vi "Start.vi"(0 "eye scan in":refnum<class "niHighSpeedSerial Eye Scan v1 Host.lvclass">, 11 "error in":errorcluster) -> (4 "eye scan out":refnum<class "niHighSpeedSerial Eye Scan v1 Host.lvclass">, 15 "error out":errorcluster)   [LabVIEW 2014, in "niHighSpeedSerial Eye Scan v1 Host.lvclass"]
doc: "Moves the session into the Running state and begins measuring the first point.\n\n<B>Input Parameters</B>\n\n<B>eye scan in</B> Takes in a reference to your session from the previous VI.\n\n<B>error in</B> describes error conditions that occur before this node runs. This input provides standard 'error in' functionality.\n\n<B>Output Parameters</B>\n\n<B>eye scan out</B> passes a reference to your session to the next VI.\n\n<B>error out</B> contains error information. This output provides standard 'error out' functionality."
uses:
  <instrlib>/niHighSpeedSerial/Eye Scan/v1/Host/Eye Scan/niHighSpeedSerial Eye Scan v1 Host.lvclass
  <instrlib>/niHighSpeedSerial/Eye Scan/v1/Host/Eye Scan/niHighSpeedSerial Eye Scan v1 Host.lvclass/niHighSpeedSerial Eye Scan v1 Host.ctl
  <instrlib>/niHighSpeedSerial/Eye Scan/v1/Host/Eye Scan/Private/Measure State.ctl
  <vilib>/Utility/error.llb/Error Cluster From Error Code.vi
  <vilib>/ErrorRing/Error Ring.xnode
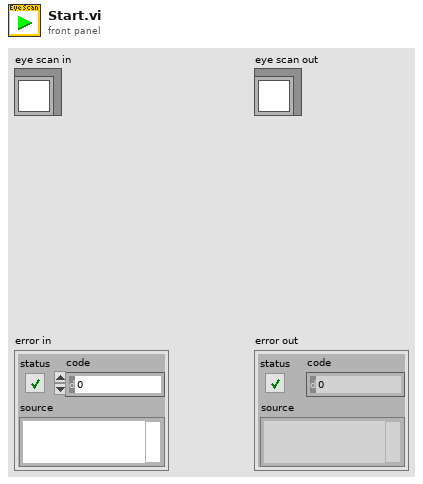
[diagram p1: front panel]
types:
  T1 = typedef "niHighSpeedSerial Eye Scan v1 Host.lvclass/Measure State.ctl" = enum16{"Uninitialized", "Initialized", "Ready", "Measuring", "Finished", "Aborted"}
  T2 = typedef "niHighSpeedSerial Eye Scan v1 Host.lvclass/Private Data.ctl" = cluster{"instruction target":refnum<class "niInstr Instruction Target v1 Host.lvclass">, "channels":T3[], "measure state":T1, "rx output divider":T4, "equalization mode":T5, "rx data width":T6, "BER floor":dbl, "number of points completed":i32, "rx output divider configured?":bool, "equalization mode configured?":bool, "rx data width configured?":bool}
  T3 = typedef "niHighSpeedSerial Eye Scan v1 Host.lvclass/Channel Data.ctl" = cluster{"instance":u8, "channel":refnum<class "niHighSpeedSerial Eye Scan Single Point v1 Host.lvclass">, "point iterator":refnum<class "niHighSpeedSerial Eye Scan Point Iterator v1 Host.lvclass">}
  T4 = typedef "niHighSpeedSerial Eye Scan Common v1 Host.lvlib/RX Output Divider.ctl" = enum16{"1", "2", "4", "8", "16"}
  T5 = typedef "niHighSpeedSerial Eye Scan Common v1 Host.lvlib/Equalization Mode.ctl" = enum16{"DFE", "LPM"}
  T6 = typedef "niHighSpeedSerial Eye Scan Common v1 Host.lvlib/Data Width.ctl" = enum16{"16 Bit", "20 Bit", "32 Bit", "40 Bit"}
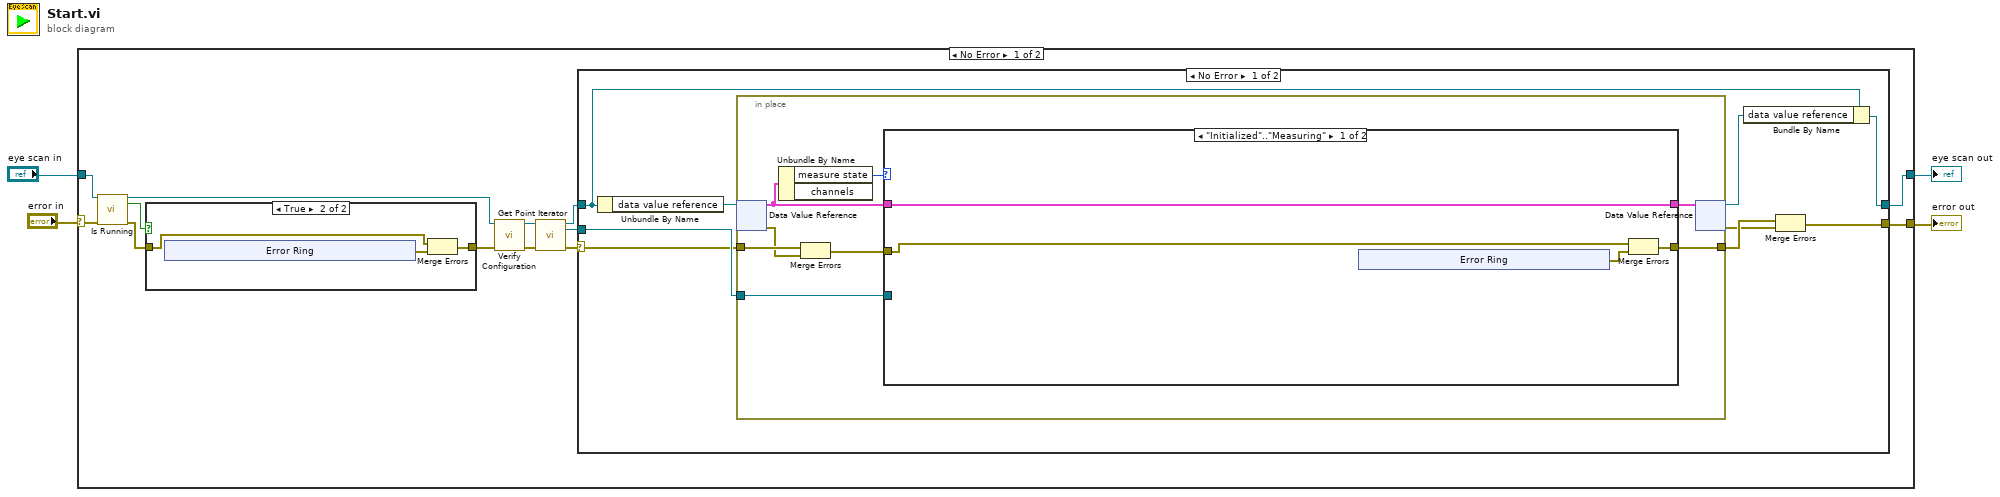
[diagram p0: block diagram]
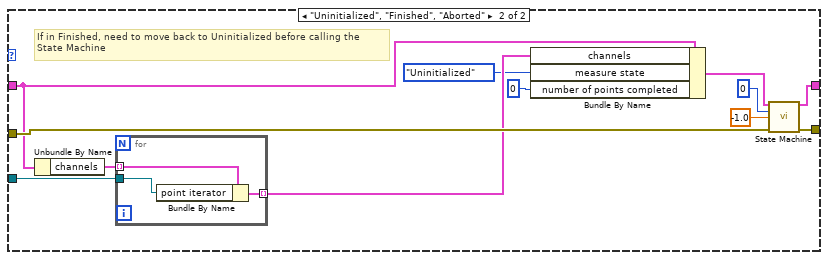
[diagram p3: hidden frame]
diagram:
  n1 = case shown="No Error" "error in" {
    selector: "error in" -> [w9 w69]
    tunnel: [w17 w69] -> w3
    tunnel: "eye scan in" -> [w10 w68]
    tunnel: [w16 w68] -> w1
    frame No Error {
      n2 = call <instrlib>:"Is Running.vi"("eye scan in"=w10, "error in"=w9) -> ("eye scan out"=w8:refnum<class "niHighSpeedSerial Eye Scan v1 Host.lvclass">, "is running?"=w6:bool, "error out"=w5:errorcluster)  [unwired: 11 in]
      n3 = case shown="True" w6 {
        tunnel: w5 -> [w18 w21]
        tunnel: [w18 w20] -> w7
        frame False {
        }
        frame True {
          n4 = xnode "Error Ring"() -> ("error out"=w19:errorcluster)
          n5 = Merge Errors(w21, w19) -> (w20:errorcluster)
        }
      }
      n6 = call-dynamic "Verify Configuration.vi"("eye scan in"=w8, "error in"=w7) -> ("eye scan out"=w11:refnum<class "niHighSpeedSerial Eye Scan v1 Host.lvclass">, "error out"=w13:errorcluster)  [unwired: 12 in]
      n7 = call-dynamic "Get Point Iterator.vi"("eye scan in"=w11, "error in"=w13) -> ("eye scan out"=w15:refnum<class "niHighSpeedSerial Eye Scan v1 Host.lvclass">, "eye scan point iterator"=w14:refnum<class "niHighSpeedSerial Eye Scan Point Iterator v1 Host.lvclass">, "error out"=w12:errorcluster)  [unwired: 11 in]
      n8 = case shown="No Error" w12 {
        selector: w12 -> [w26 w67]
        tunnel: [w31 w67] -> w17
        tunnel: [w29 w66] -> w16
        tunnel: w15 -> [w28 w66]
        tunnel: w14 -> [w27 _]
        frame No Error {
          n9 = Unbundle By Name(w28) -> ("data value reference"=w34:refnum<data-value>)
          n10 = in-place {
            in-place-border: w26 -> [w42]
            in-place-border: [w38] -> w33
            in-place-border: w27 -> [w35]
            n11 = in-place-dvr #1(w34) -> (w37:T2, w41:errorcluster)
            n12 = Unbundle By Name(w37) -> ("measure state"=w36:T1)  [unwired: 1 out]
            n13 = Merge Errors(w42, w41) -> (w39:errorcluster)
            n14 = case shown="\"Initialized\"..\"Measuring\"" w36 {
              tunnel: [w46 w62] -> w40
              tunnel: w39 -> [w45 w59]
              tunnel: [w43 w61] -> w38
              tunnel: w37 -> [w46 w57]
              tunnel: w35 -> [_ w60]
              frame "Initialized".."Measuring" {
                n15 = xnode "Error Ring"() -> ("error out"=w44:errorcluster)
                n16 = Merge Errors(w45, w44) -> (w43:errorcluster)
              }
              frame "Uninitialized", "Finished", "Aborted" {
                # "If in Finished, need to move back to Uninitialized before calling the\nState Machine"
                n17 = Unbundle By Name(w57) -> ("channels"=w58:T3[])
                n18 = for {
                  tunnel: w60 -> [w64]
                  tunnel: w58 -> [w65] mode=indexing
                  tunnel: [w63] -> w55 mode=indexing
                  n19 = Bundle By Name(cluster=w65, "point iterator"=w64) -> (w63:T3)
                }
                n20 = Bundle By Name(cluster=w57, "channels"=w55, "measure state"=Measure_State."Uninitialized" ("Measure State"), "number of points completed"=0) -> (w56:T2)
                n21 = call <instrlib>:"State Machine.vi"("private data"=w56, "requested number of new points"=0 ("Requested Number of Points"), "timeout (100 ms)"=-1.0 ("Timeout (100 ms)"), "error in"=w59) -> ("private data out"=w62:T2, "error out"=w61:errorcluster)  [unwired: 7 in, 3 out]
              }
            }
            n22 = in-place-dvr #1(w40) -> (w30:refnum<data-value>, w32:errorcluster)
          }
          n23 = Bundle By Name(cluster=w28, "data value reference"=w30) -> (w29:refnum<class "niHighSpeedSerial Eye Scan v1 Host.lvclass">)
          n24 = Merge Errors(w33, w32) -> (w31:errorcluster)
        }
        frame Error {
        }
      }
    }
    frame Error {
    }
  }
  "error out" <- w3
  "eye scan out" <- w1
